vi "arrayfrom0to255.vi"() -> (3 "Array 2":i32[](array[numeric]))   [LabVIEW 2013]
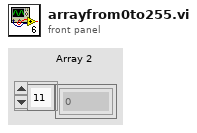
[diagram p1: front panel]
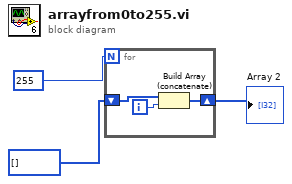
[diagram p0: block diagram]
diagram:
  n1 = for {
    N: 255 -> [_]
    shift-right: [w4] -> w2
    shift-left: i32[] [] -> [w6]
    i -> [w5]
    n2 = Build Array (concatenate)(w6, w5) -> (w4:i32[])
  }
  "Array 2" <- w2
